vi "escribe_final_ajustes_previos.vi"(8 "error in (no error)":errorcluster, 10 "Datos a Escribir":T1={"igualacion_de_patrones"={"Nivel Emitido Pistófono [dB]"=0.0, "Temperatura interna Pistófono[ºC]"=0.0, "Presión Medida Pistófono  [hPa]"=0.0, "Humedad Relativa Aire [%]"=0.0, "Factor de corrección de sensibilidad Nexus"=0.0}, "Tabla Referencia Acústica Generador Externo"=[], "Voltaje enviado a CAM"=0.0, "usuario_registra"=1, "id_pon_frecuencia"=0}, 11 "DB in":refnum<class "Base de Datos.lvclass">) -> (0 "error out":errorcluster, 3 "DB out":refnum<class "Base de Datos.lvclass">)   [LabVIEW 2019, in "Base de Datos.lvclass"]
uses:
  Base de Datos.lvclass
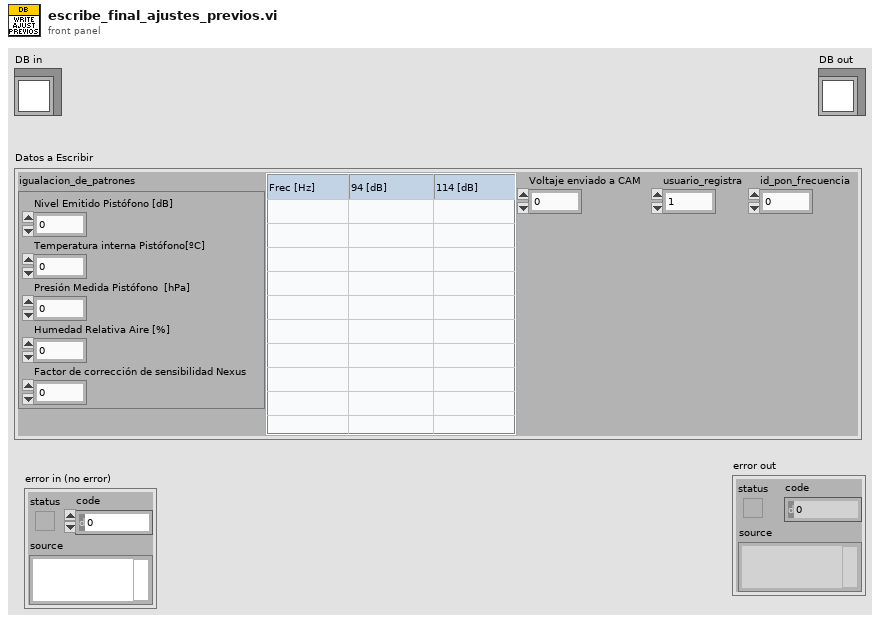
[diagram p1: front panel]
types:
  T1 = cluster{"igualacion_de_patrones":cluster{"Nivel Emitido Pistófono [dB]":dbl, "Temperatura interna Pistófono[ºC]":dbl, "Presión Medida Pistófono  [hPa]":dbl, "Humedad Relativa Aire [%]":dbl, "Factor de corrección de sensibilidad Nexus":dbl}, "Tabla Referencia Acústica Generador Externo":string[][], "Voltaje enviado a CAM":dbl, "usuario_registra":i32, "id_pon_frecuencia":i32}
  T2 = cluster{"Nivel Emitido Pistófono [dB]":dbl, "Temperatura interna Pistófono[ºC]":dbl, "Presión Medida Pistófono  [hPa]":dbl, "Humedad Relativa Aire [%]":dbl, "Factor de corrección de sensibilidad Nexus":dbl}
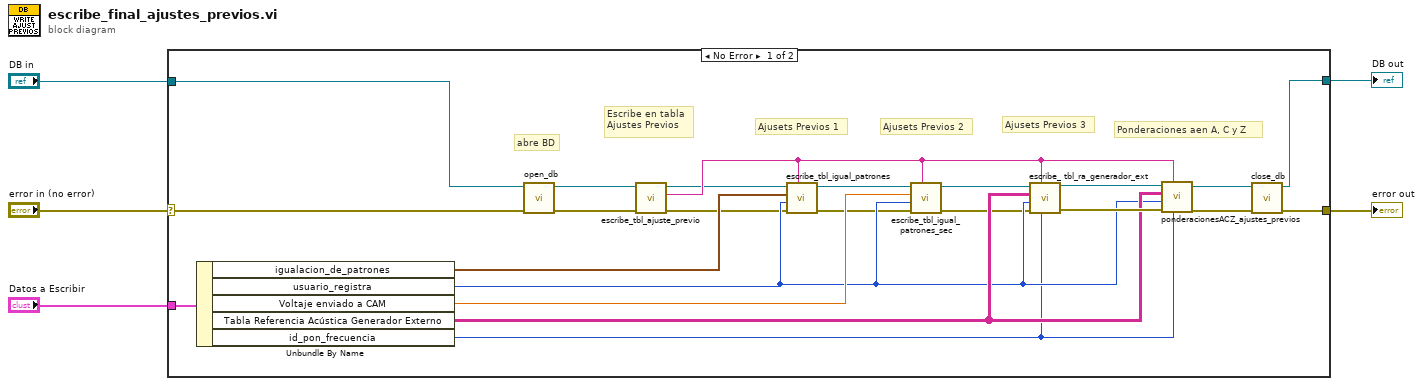
[diagram p0: block diagram]
diagram:
  n1 = case shown="No Error" "error in (no error)" {
    selector: "error in (no error)" -> [w27 w30]
    tunnel: [w28 w30] -> w5
    tunnel: "DB in" -> [w26 w29]
    tunnel: [w25 w29] -> w2
    tunnel: "Datos a Escribir" -> [w24 _]
    frame No Error {
      # "Ponderaciones aen A, C y Z"
      # "abre BD"
      # "Ajusets Previos 3"
      # "Ajusets Previos 2"
      # "Ajusets Previos 1"
      # "Escribe en tabla \nAjustes Previos"
      n2 = Unbundle By Name(w24) -> ("igualacion_de_patrones"=w23:T2, "usuario_registra"=w15:i32, "Voltaje enviado a CAM"=w22:dbl, "Tabla Referencia Acústica Generador Externo"=w17:string[][], "id_pon_frecuencia"=w14:i32)
      n3 = call "open_db.vi"("error in (no error)"=w27, "DB in"=w26) -> ("error out"=w12:errorcluster, "DB out"=w13:refnum<class "Base de Datos.lvclass">)  [unwired: 8 in]
      n4 = call "escribe_tbl_ajuste_previo.vi"("error in (no error)"=w12, "DB in"=w13) -> ("error out"=w10:errorcluster, "last_id_ajuste_previo"=w16:string, "object out"=w11:refnum<class "Base de Datos.lvclass">)  [unwired: 7 in]
      n5 = call "escribe_tbl_igual_patrones.vi"("last_id_ajuste_previo"=w16, "error in (no error)"=w10, "usuario_registra"=w15, "igualacion_de_patrones"=w23, "DB in"=w11) -> ("error out"=w8:errorcluster, "DB out"=w9:refnum<class "Base de Datos.lvclass">)  [unwired: 5 in]
      n6 = call "escribe_tbl_igual_patrones_sec.vi"("last_id_ajuste_previo"=w16, "error in (no error)"=w8, "usuario_registra"=w15, "Voltaje enviado a CAM"=w22, "BD in"=w9) -> ("error out"=w6:errorcluster, "BD out"=w7:refnum<class "Base de Datos.lvclass">)  [unwired: 5 in]
      n7 = call "escribe_ tbl_ra_generador_ext.vi"("id_pon_frecuencia"=w14, "last_id_ajuste_previo"=w16, "error in (no error)"=w6, "usuario_registra"=w15, "Tabla Referencia Acústica Generador Externo"=w17, "BD in"=w7) -> ("error out"=w20:errorcluster, "BD out"=w21:refnum<class "Base de Datos.lvclass">)  [unwired: 4 in]
      n8 = call "ponderacionesACZ_ajustes_previos.vi"("id_pon_frecuencia"=w14, "last_id_ajuste_previo"=w16, "error in (no error)"=w20, "usuario_registra"=w15, "Tabla Referencia Acústica Generador Externo"=w17, "BD in"=w21) -> ("error out"=w18:errorcluster, "BD out"=w19:refnum<class "Base de Datos.lvclass">)  [unwired: 4 in]
      n9 = call "close_db.vi"("error in (no error)"=w18, "BD in"=w19) -> ("error out"=w28:errorcluster, "BD out"=w25:refnum<class "Base de Datos.lvclass">)  [unwired: 8 in]
    }
    frame Error {
    }
  }
  "error out" <- w5
  "DB out" <- w2
